vi "Initialize.vi"(8 "Error In":errorcluster, 9 "Tolerance (m)":dbl, 10 "Drive Location":T1 {"North" format="%#_10f"; "East" format="%#_8f"}) -> (0 "Error Out":errorcluster, 3 "Drive out":refnum<class "DriveTo.lvclass">)   [LabVIEW 2011, in "DriveTo.lvclass"]
uses:
  DriveTo.lvclass
  2 Typedefs/UTM Location.ctl
  DriveTo.lvclass/DriveTo.ctl
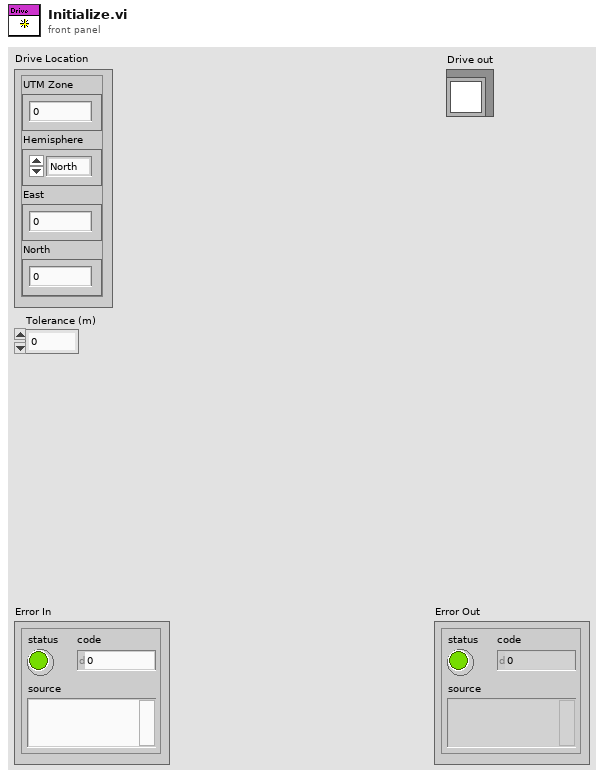
[diagram p1: front panel]
types:
  T1 = typedef "UTM Location.ctl" = cluster{"UTM Zone":dbl, "Hemisphere":enum16{"North", "South"}, "East":dbl, "North":dbl}
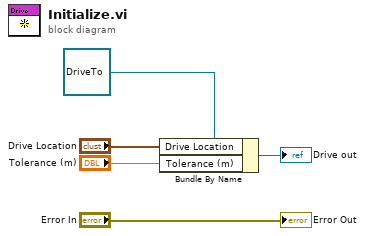
[diagram p0: block diagram]
diagram:
  n1 = Bundle By Name(cluster=refnum<class "DriveTo.lvclass"> refnum ("PassBuoys in"), "Drive Location"="Drive Location", "Tolerance (m)"="Tolerance (m)") -> (→"Drive out":refnum<class "DriveTo.lvclass">)
  "Error Out" <- "Error In"
